vi "Check If Error Exists.vi"(8 "error in":errorcluster, 10 "error key":string, 11 "ni-switch custom device in":T1 format="%.0x") -> (0 "error out":errorcluster, 2 "error exists?":bool, 3 "ni-switch custom device out":T1 format="%.0x")   [LabVIEW 2017, in "NI-SWITCH System Explorer.lvlib"]
uses:
  NI-SWITCH System Explorer.lvlib
  <vilib>/NI Veristand/Custom Device API/Custom Device Item Ref.ctl
  NationalInstruments.VeriStand.SystemDefinitionAPI
  NationalInstruments.VeriStand.SystemStorage
  <vilib>/NI VeriStand/Custom Device API/Custom Device API.lvlib
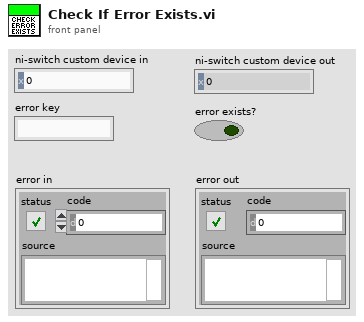
[diagram p1: front panel]
types:
  T1 = typedef "Custom Device API.lvlib/Custom Device Item Ref.ctl" = u64
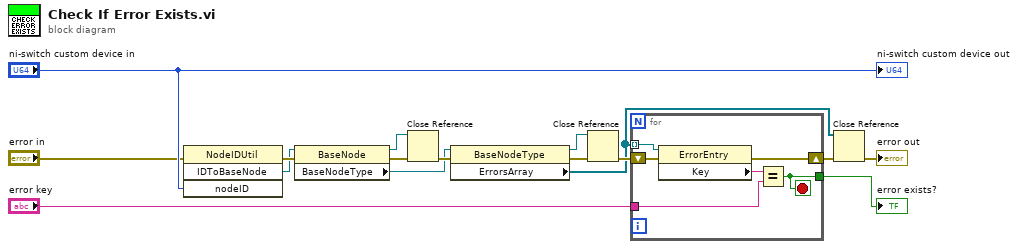
[diagram p0: block diagram]
diagram:
  n1 = invoke class="NodeIDUtil" method="IDToBaseNode"(error in="error in", "nodeID"="ni-switch custom device in") -> (error out=w7:errorcluster, "IDToBaseNode"=w2:refnum<k24>)  [unwired: 2 in, 2 out]
  n2 = property class="BaseNode"(reference=w2, error in=w7) -> (reference out=w13:refnum<k24>, error out=w6:errorcluster, "BaseNodeType"=w3:refnum<k24>)
  n3 = Close Reference(reference=w13, error in (no error)=w6) -> (error out=w12:errorcluster)
  n4 = property class="BaseNodeType"(reference=w3, error in=w12) -> (reference out=w15:refnum<k24>, error out=w5:errorcluster, "ErrorsArray"=w8:refnum<k24>[])
  n5 = Close Reference(reference=w15, error in (no error)=w5) -> (error out=w14:errorcluster)
  n6 = for {
    tunnel: w8 -> [w22] mode=indexing
    shift-right: [w21] -> w4
    shift-left: w14 -> [w20]
    tunnel: "error key" -> [w18]
    tunnel: [w17] -> w9
    stop <- w17 stop-if-true
    n7 = property class="ErrorEntry"(reference=w22, error in=w20) -> (error out=w21:errorcluster, "Key"=w19:string)  [unwired: 1 out]
    n8 = Equal?(x=w19, y=w18) -> (x = y?=w17:bool)
  }
  "error exists?" <- w9
  n9 = Close Reference(reference=w8, error in (no error)=w4) -> (error out=→"error out":errorcluster)
  "ni-switch custom device out" <- "ni-switch custom device in"
